vi "Target3.vi"   [LabVIEW 2025]
uses:
  <vilib>/eio/utilities/niEioResolveVilibRelativePath.vi
  <vilib>/rvi/interface/RandomDataEmulation/niFpgaRandomDataHandleErrors.vi
  <vilib>/rvi/Memory/Memory_Emulation/nirvimemoryFastEmulation.vi
  <vilib>/rvi/Memory/Memory_Emulation/nirvimemoryEmulation.vi
  <vilib>/rvi/Emulation/niFpgaEmulationIsFPGAContextNoSignature.vi
  <vilib>/rvi/DataTransferAndStorage/Container/Common/niFpgaContainerGetUniqueNameForEmu.vi
  <vilib>/rvi/Emulation/niFpgaProcessEmulError.vi
  <vilib>/rvi/Emulation/niFpgaSctlEmulationGetInTimedLoop.vi
  <vilib>/rvi/errors/nirviReportUnexpectedCaseInternalError (U32).vi
  <vilib>/rvi/DataTransferAndStorage/Container/XNode/niFpgaContainer.xnode
  <vilib>/rvi/interface/RandomDataEmulation/nirviRandomDataFpgaReadWriteTemplate.vi
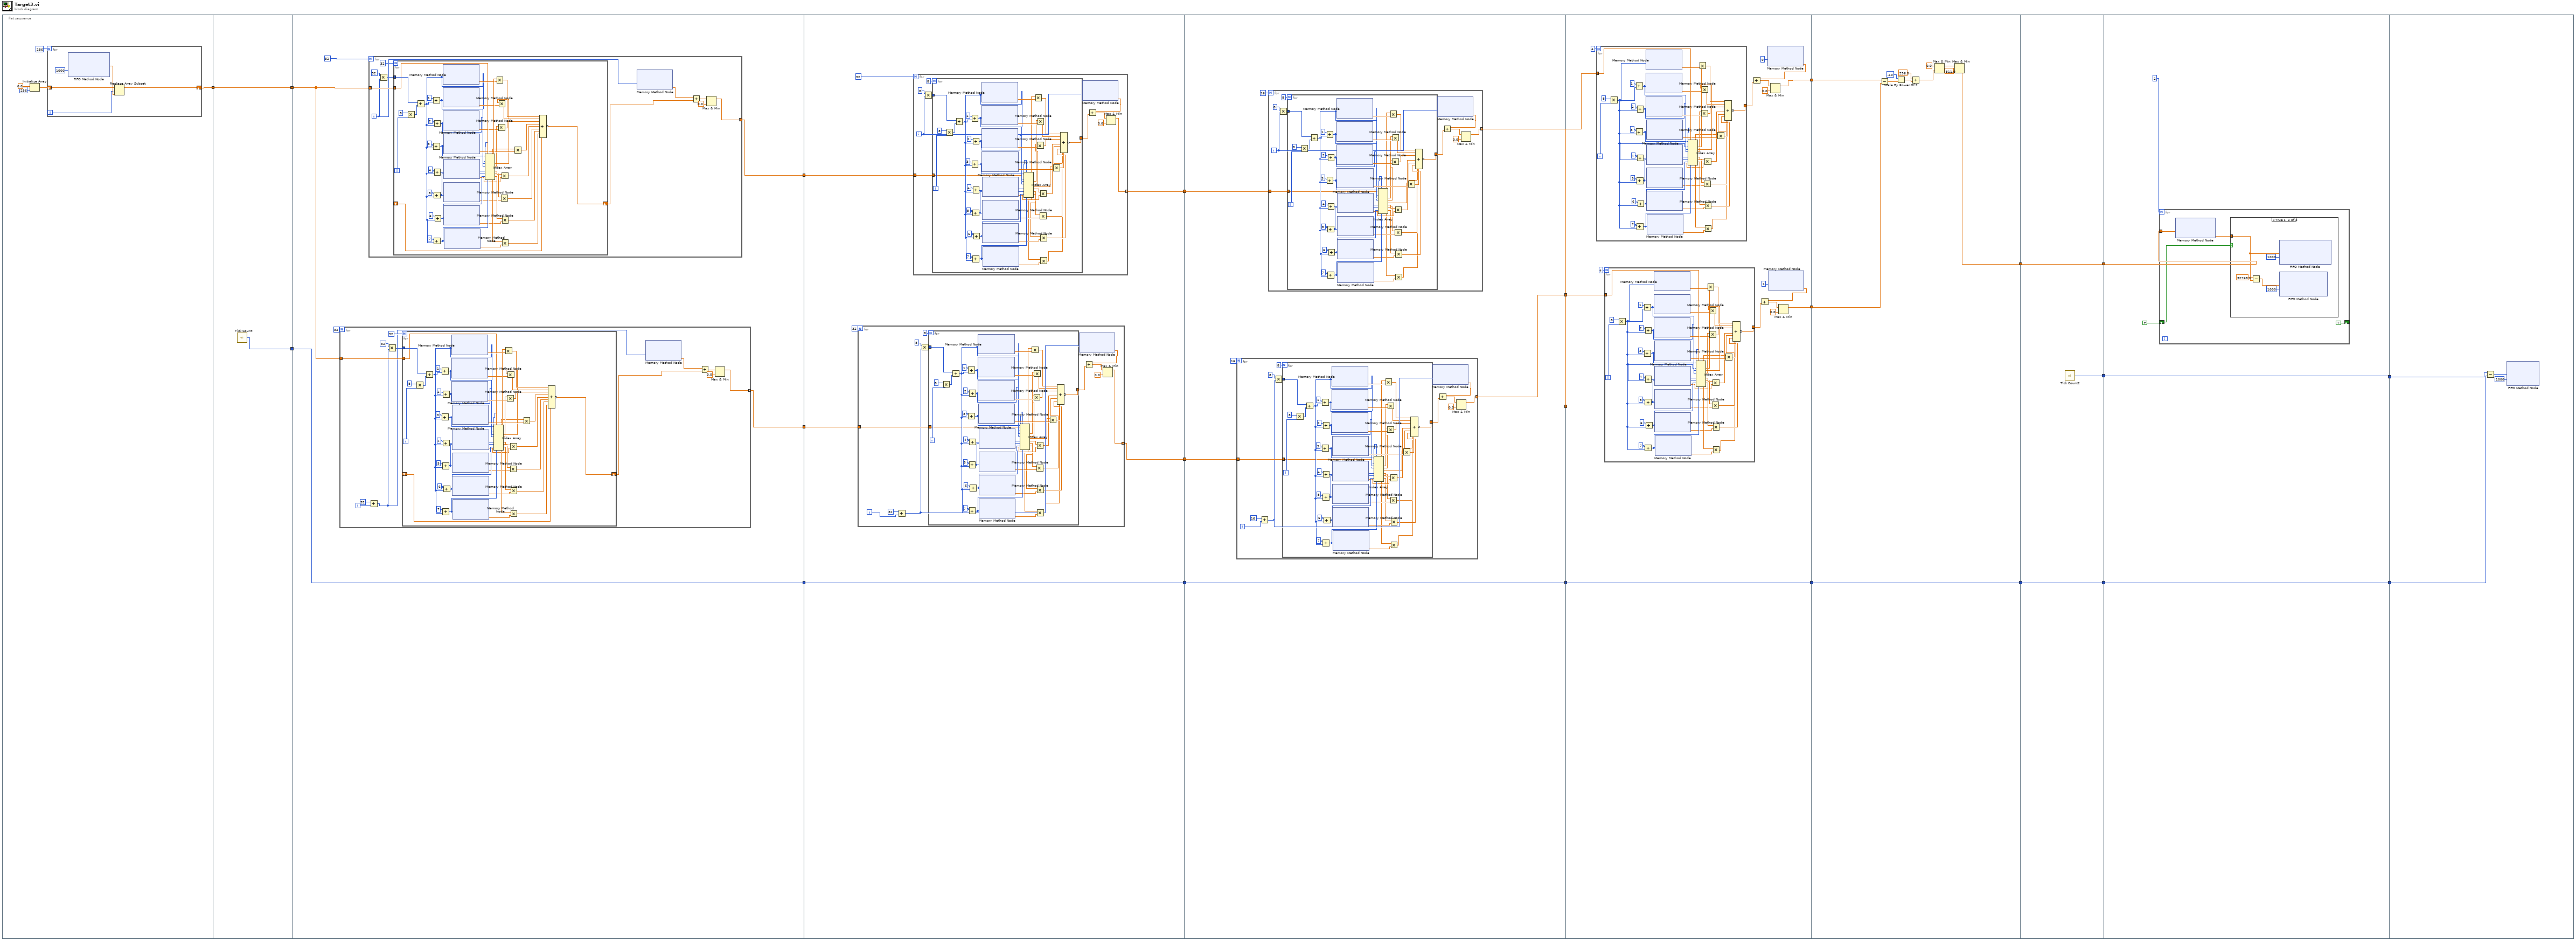
[diagram p0: block diagram]
diagram:
  n1 = flat-sequence {
    tunnel: [w26] -> w22
    tunnel: w22 -> [w34]
    tunnel: [w34] -> w21
    tunnel: [w33] -> w20
    tunnel: w21 -> [w36]
    tunnel: w20 -> [w39]
    tunnel: [w39] -> w10
    tunnel: [w38] -> w9
    tunnel: [w35] -> w2
    tunnel: w10 -> [w161]
    tunnel: [w161] -> w7
    tunnel: w9 -> [w159]
    tunnel: [w158] -> w5
    tunnel: w2 -> [w156]
    tunnel: [w155] -> w1
    tunnel: [w278] -> w8
    tunnel: w7 -> [w280]
    tunnel: [w280] -> w6
    tunnel: w5 -> [w277]
    tunnel: [w276] -> w3
    tunnel: w1 -> [w274]
    tunnel: w8 -> [w408]
    tunnel: [w407] -> w19
    tunnel: [w409] -> w11
    tunnel: w6 -> [w409]
    tunnel: [w394] -> w4
    tunnel: w3 -> [w393]
    tunnel: w19 -> [w496]
    tunnel: [w499] -> w18
    tunnel: [w498] -> w12
    tunnel: w11 -> [w498]
    tunnel: w4 -> [w497]
    tunnel: w18 -> [w510]
    tunnel: [w510] -> w17
    tunnel: [w509] -> w16
    tunnel: [w508] -> w13
    tunnel: w12 -> [w508]
    tunnel: w17 -> [w514]
    tunnel: [w512] -> w15
    tunnel: w16 -> [w512]
    tunnel: [w511] -> w14
    tunnel: w13 -> [w511]
    tunnel: w15 -> [w528]
    tunnel: w14 -> [w525]
    frame #0 {
      n2 = Initialize Array(sgl 0.0 ("element"), 256 ("dimension size")) -> (w23:sgl[])
      n3 = for {
        N: 256 -> [_]
        shift-right: [w29] -> w26
        shift-left: w23 -> [w31]
        i -> [w28]
        n4 = xnode ("FIFO Method Node")("Timeout"=1000) -> ("Element"=w30:sgl)  [unwired: 1 in, 2 out]
        n5 = Replace Array Subset(array=w31, new element=w30, index=w28) -> (w29:sgl[])
      }
    }
    frame #1 {
      n6 = call "Tick Count"() -> ("Tick Count(uSec)"=w33:u32)
    }
    frame #2 {
      n7 = for {
        N: 32 -> [_]
        tunnel: w36 -> [w47]
        tunnel: [w46] -> w35 mode=indexing
        i -> [w43]
        n8 = Add(x=32, y=w43) -> (x+y=w42:i32)
        n9 = Multiply(x=32, y=w42) -> (x*y=w50:i32)
        n10 = for {
          N: 32 -> [_]
          tunnel: w50 -> [w98]
          tunnel: w47 -> [w84]
          shift-right: [w53] -> w45
          shift-left: _ -> [w54]
          i -> [w97]
          n11 = Multiply(x=8, y=w97) -> (x*y=w95:i32)
          n12 = Add(x=w98, y=w95) -> (x+y=w59:i32)
          n13 = Add(x=1, y=w59) -> (x+y=w81:i32)
          n14 = Add(x=3, y=w59) -> (x+y=w77:i32)
          n15 = Add(x=5, y=w59) -> (x+y=w70:i32)
          n16 = Add(x=7, y=w59) -> (x+y=w68:i32)
          n17 = Add(x=2, y=w59) -> (x+y=w76:i32)
          n18 = Add(x=4, y=w59) -> (x+y=w71:i32)
          n19 = Add(x=6, y=w59) -> (x+y=w69:i32)
          n20 = xnode ("Memory Method Node")("Address"=w59) -> ("Data"=w90:sgl)  [unwired: 1 in, 1 out]
          n21 = xnode ("Memory Method Node")("Address"=w81) -> ("Data"=w85:sgl)  [unwired: 1 in, 1 out]
          n22 = xnode ("Memory Method Node")("Address"=w76) -> ("Data"=w82:sgl)  [unwired: 1 in, 1 out]
          n23 = xnode ("Memory Method Node")("Address"=w77) -> ("Data"=w83:sgl)  [unwired: 1 in, 1 out]
          n24 = xnode ("Memory Method Node")("Address"=w71) -> ("Data"=w60:sgl)  [unwired: 1 in, 1 out]
          n25 = xnode ("Memory Method Node")("Address"=w70) -> ("Data"=w61:sgl)  [unwired: 1 in, 1 out]
          n26 = xnode ("Memory Method Node")("Address"=w69) -> ("Data"=w62:sgl)  [unwired: 1 in, 1 out]
          n27 = xnode ("Memory Method Node")("Address"=w68) -> ("Data"=w63:sgl)  [unwired: 1 in, 1 out]
          n28 = Index Array(array=w84, index #1=w59, index #2=w81, index #3=w76, index #4=w77, index #5=w71, index #6=w70, index #7=w69, index #8=w68) -> (element #1=w91:sgl, element #2=w80:sgl, element #3=w79:sgl, element #4=w78:sgl, element #5=w67:sgl, element #6=w66:sgl, element #7=w65:sgl, element #8=w64:sgl)
          n29 = Multiply(x=w91, y=w90) -> (x*y=w89:sgl)
          n30 = Multiply(x=w79, y=w82) -> (x*y=w87:sgl)
          n31 = Multiply(x=w80, y=w85) -> (x*y=w88:sgl)
          n32 = Multiply(x=w66, y=w61) -> (x*y=w57:sgl)
          n33 = Multiply(x=w67, y=w60) -> (x*y=w58:sgl)
          n34 = Multiply(x=w65, y=w62) -> (x*y=w56:sgl)
          n35 = Multiply(x=w64, y=w63) -> (x*y=w55:sgl)
          n36 = Multiply(x=w78, y=w83) -> (x*y=w86:sgl)
          n37 = Compound Arithmetic op=ADD(w89, w88, w87, w86, w58, w57, w56, w55, w54) -> (invert w53:sgl)
        }
        n38 = xnode ("Memory Method Node")("Address"=w42) -> ("Data"=w44:sgl)  [unwired: 1 in, 1 out]
        n39 = Add(x=w44, y=w45) -> (x+y=w49:sgl)
        n40 = Max & Min(x=w49, y=sgl 0.0) -> (max(x,y)=w46:sgl)  [unwired: 1 out]
      }
      n41 = for {
        N: 32 -> [_]
        tunnel: w36 -> [w103]
        tunnel: [w101] -> w38 mode=indexing
        i -> [w102]
        n42 = Multiply(x=32, y=w102) -> (x*y=w106:i32)
        n43 = for {
          N: 32 -> [_]
          tunnel: w106 -> [w154]
          tunnel: w103 -> [w140]
          shift-right: [w109] -> w100
          shift-left: _ -> [w110]
          i -> [w153]
          n44 = Multiply(x=8, y=w153) -> (x*y=w151:i32)
          n45 = Add(x=w154, y=w151) -> (x+y=w115:i32)
          n46 = Add(x=1, y=w115) -> (x+y=w137:i32)
          n47 = Add(x=3, y=w115) -> (x+y=w133:i32)
          n48 = Add(x=5, y=w115) -> (x+y=w126:i32)
          n49 = Add(x=7, y=w115) -> (x+y=w124:i32)
          n50 = Add(x=2, y=w115) -> (x+y=w132:i32)
          n51 = Add(x=4, y=w115) -> (x+y=w127:i32)
          n52 = Add(x=6, y=w115) -> (x+y=w125:i32)
          n53 = xnode ("Memory Method Node")("Address"=w115) -> ("Data"=w146:sgl)  [unwired: 1 in, 1 out]
          n54 = xnode ("Memory Method Node")("Address"=w137) -> ("Data"=w141:sgl)  [unwired: 1 in, 1 out]
          n55 = xnode ("Memory Method Node")("Address"=w132) -> ("Data"=w138:sgl)  [unwired: 1 in, 1 out]
          n56 = xnode ("Memory Method Node")("Address"=w133) -> ("Data"=w139:sgl)  [unwired: 1 in, 1 out]
          n57 = xnode ("Memory Method Node")("Address"=w127) -> ("Data"=w116:sgl)  [unwired: 1 in, 1 out]
          n58 = xnode ("Memory Method Node")("Address"=w126) -> ("Data"=w117:sgl)  [unwired: 1 in, 1 out]
          n59 = xnode ("Memory Method Node")("Address"=w125) -> ("Data"=w118:sgl)  [unwired: 1 in, 1 out]
          n60 = xnode ("Memory Method Node")("Address"=w124) -> ("Data"=w119:sgl)  [unwired: 1 in, 1 out]
          n61 = Index Array(array=w140, index #1=w115, index #2=w137, index #3=w132, index #4=w133, index #5=w127, index #6=w126, index #7=w125, index #8=w124) -> (element #1=w147:sgl, element #2=w136:sgl, element #3=w135:sgl, element #4=w134:sgl, element #5=w123:sgl, element #6=w122:sgl, element #7=w121:sgl, element #8=w120:sgl)
          n62 = Multiply(x=w147, y=w146) -> (x*y=w145:sgl)
          n63 = Multiply(x=w135, y=w138) -> (x*y=w143:sgl)
          n64 = Multiply(x=w136, y=w141) -> (x*y=w144:sgl)
          n65 = Multiply(x=w122, y=w117) -> (x*y=w113:sgl)
          n66 = Multiply(x=w123, y=w116) -> (x*y=w114:sgl)
          n67 = Multiply(x=w121, y=w118) -> (x*y=w112:sgl)
          n68 = Multiply(x=w120, y=w119) -> (x*y=w111:sgl)
          n69 = Multiply(x=w134, y=w139) -> (x*y=w142:sgl)
          n70 = Compound Arithmetic op=ADD(w145, w144, w143, w142, w114, w113, w112, w111, w110) -> (invert w109:sgl)
        }
        n71 = xnode ("Memory Method Node")("Address"=w102) -> ("Data"=w99:sgl)  [unwired: 1 in, 1 out]
        n72 = Add(x=w99, y=w100) -> (x+y=w105:sgl)
        n73 = Max & Min(x=w105, y=sgl 0.0) -> (max(x,y)=w101:sgl)  [unwired: 1 out]
      }
    }
    frame #3 {
      n74 = for {
        N: 32 -> [_]
        tunnel: w156 -> [w166]
        tunnel: [w165] -> w155 mode=indexing
        i -> [w163]
        n75 = Add(x=32, y=w163) -> (x+y=w162:i32)
        n76 = Multiply(x=8, y=w162) -> (x*y=w170:i32)
        n77 = for {
          N: 8 -> [_]
          tunnel: w170 -> [w218]
          tunnel: [w203] -> w167
          tunnel: w166 -> [w182]
          i -> [w217]
          n78 = Multiply(x=8, y=w217) -> (x*y=w215:i32)
          n79 = Add(x=w218, y=w215) -> (x+y=w183:i32)
          n80 = Add(x=1, y=w183) -> (x+y=w202:i32)
          n81 = Add(x=3, y=w183) -> (x+y=w201:i32)
          n82 = Add(x=5, y=w183) -> (x+y=w194:i32)
          n83 = Add(x=7, y=w183) -> (x+y=w192:i32)
          n84 = Add(x=2, y=w183) -> (x+y=w200:i32)
          n85 = Add(x=4, y=w183) -> (x+y=w195:i32)
          n86 = Add(x=6, y=w183) -> (x+y=w193:i32)
          n87 = xnode ("Memory Method Node")("Address"=w183) -> ("Data"=w211:sgl)  [unwired: 1 in, 1 out]
          n88 = xnode ("Memory Method Node")("Address"=w202) -> ("Data"=w206:sgl)  [unwired: 1 in, 1 out]
          n89 = xnode ("Memory Method Node")("Address"=w200) -> ("Data"=w204:sgl)  [unwired: 1 in, 1 out]
          n90 = xnode ("Memory Method Node")("Address"=w201) -> ("Data"=w205:sgl)  [unwired: 1 in, 1 out]
          n91 = xnode ("Memory Method Node")("Address"=w195) -> ("Data"=w188:sgl)  [unwired: 1 in, 1 out]
          n92 = xnode ("Memory Method Node")("Address"=w194) -> ("Data"=w189:sgl)  [unwired: 1 in, 1 out]
          n93 = xnode ("Memory Method Node")("Address"=w193) -> ("Data"=w190:sgl)  [unwired: 1 in, 1 out]
          n94 = xnode ("Memory Method Node")("Address"=w192) -> ("Data"=w191:sgl)  [unwired: 1 in, 1 out]
          n95 = Index Array(array=w182, index #1=w183, index #2=w202, index #3=w200, index #4=w201, index #5=w195, index #6=w194, index #7=w193, index #8=w192) -> (element #1=w181:sgl, element #2=w180:sgl, element #3=w179:sgl, element #4=w177:sgl, element #5=w178:sgl, element #6=w176:sgl, element #7=w175:sgl, element #8=w174:sgl)
          n96 = Multiply(x=w181, y=w211) -> (x*y=w210:sgl)
          n97 = Multiply(x=w179, y=w204) -> (x*y=w208:sgl)
          n98 = Multiply(x=w180, y=w206) -> (x*y=w209:sgl)
          n99 = Multiply(x=w176, y=w189) -> (x*y=w186:sgl)
          n100 = Multiply(x=w178, y=w188) -> (x*y=w187:sgl)
          n101 = Multiply(x=w175, y=w190) -> (x*y=w185:sgl)
          n102 = Multiply(x=w174, y=w191) -> (x*y=w184:sgl)
          n103 = Multiply(x=w177, y=w205) -> (x*y=w207:sgl)
          n104 = Compound Arithmetic op=ADD(w210, w209, w208, w207, w187, w186, w185, w184) -> (invert w203:sgl)
        }
        n105 = xnode ("Memory Method Node")("Address"=w162) -> ("Data"=w172:sgl)  [unwired: 1 in, 1 out]
        n106 = Add(x=w172, y=w167) -> (x+y=w169:sgl)
        n107 = Max & Min(x=w169, y=sgl 0.0) -> (max(x,y)=w165:sgl)  [unwired: 1 out]
      }
      n108 = for {
        N: 32 -> [_]
        tunnel: w159 -> [w220]
        tunnel: [w219] -> w158 mode=indexing
        i -> [w225]
        n109 = Multiply(x=8, y=w225) -> (x*y=w224:i32)
        n110 = for {
          N: 8 -> [_]
          tunnel: w224 -> [w273]
          tunnel: [w258] -> w221
          tunnel: w220 -> [w237]
          i -> [w272]
          n111 = Multiply(x=8, y=w272) -> (x*y=w270:i32)
          n112 = Add(x=w273, y=w270) -> (x+y=w238:i32)
          n113 = Add(x=1, y=w238) -> (x+y=w257:i32)
          n114 = Add(x=3, y=w238) -> (x+y=w256:i32)
          n115 = Add(x=5, y=w238) -> (x+y=w249:i32)
          n116 = Add(x=7, y=w238) -> (x+y=w247:i32)
          n117 = Add(x=2, y=w238) -> (x+y=w255:i32)
          n118 = Add(x=4, y=w238) -> (x+y=w250:i32)
          n119 = Add(x=6, y=w238) -> (x+y=w248:i32)
          n120 = xnode ("Memory Method Node")("Address"=w238) -> ("Data"=w266:sgl)  [unwired: 1 in, 1 out]
          n121 = xnode ("Memory Method Node")("Address"=w257) -> ("Data"=w261:sgl)  [unwired: 1 in, 1 out]
          n122 = xnode ("Memory Method Node")("Address"=w255) -> ("Data"=w259:sgl)  [unwired: 1 in, 1 out]
          n123 = xnode ("Memory Method Node")("Address"=w256) -> ("Data"=w260:sgl)  [unwired: 1 in, 1 out]
          n124 = xnode ("Memory Method Node")("Address"=w250) -> ("Data"=w243:sgl)  [unwired: 1 in, 1 out]
          n125 = xnode ("Memory Method Node")("Address"=w249) -> ("Data"=w244:sgl)  [unwired: 1 in, 1 out]
          n126 = xnode ("Memory Method Node")("Address"=w248) -> ("Data"=w245:sgl)  [unwired: 1 in, 1 out]
          n127 = xnode ("Memory Method Node")("Address"=w247) -> ("Data"=w246:sgl)  [unwired: 1 in, 1 out]
          n128 = Index Array(array=w237, index #1=w238, index #2=w257, index #3=w255, index #4=w256, index #5=w250, index #6=w249, index #7=w248, index #8=w247) -> (element #1=w236:sgl, element #2=w235:sgl, element #3=w234:sgl, element #4=w232:sgl, element #5=w233:sgl, element #6=w231:sgl, element #7=w230:sgl, element #8=w229:sgl)
          n129 = Multiply(x=w236, y=w266) -> (x*y=w265:sgl)
          n130 = Multiply(x=w234, y=w259) -> (x*y=w263:sgl)
          n131 = Multiply(x=w235, y=w261) -> (x*y=w264:sgl)
          n132 = Multiply(x=w231, y=w244) -> (x*y=w241:sgl)
          n133 = Multiply(x=w233, y=w243) -> (x*y=w242:sgl)
          n134 = Multiply(x=w230, y=w245) -> (x*y=w240:sgl)
          n135 = Multiply(x=w229, y=w246) -> (x*y=w239:sgl)
          n136 = Multiply(x=w232, y=w260) -> (x*y=w262:sgl)
          n137 = Compound Arithmetic op=ADD(w265, w264, w263, w262, w242, w241, w240, w239) -> (invert w258:sgl)
        }
        n138 = xnode ("Memory Method Node")("Address"=w225) -> ("Data"=w227:sgl)  [unwired: 1 in, 1 out]
        n139 = Add(x=w227, y=w221) -> (x+y=w223:sgl)
        n140 = Max & Min(x=w223, y=sgl 0.0) -> (max(x,y)=w219:sgl)  [unwired: 1 out]
      }
    }
    frame #4 {
      n141 = for {
        N: 16 -> [_]
        tunnel: [w286] -> w276 mode=indexing
        tunnel: w274 -> [w284]
        i -> [w281]
        n142 = Add(x=16, y=w281) -> (x+y=w282:i32)
        n143 = Multiply(x=8, y=w282) -> (x*y=w289:i32)
        n144 = for {
          N: 8 -> [_]
          tunnel: w289 -> [w337]
          tunnel: [w322] -> w285
          tunnel: w284 -> [w301]
          i -> [w336]
          n145 = Multiply(x=8, y=w336) -> (x*y=w334:i32)
          n146 = Add(x=w337, y=w334) -> (x+y=w302:i32)
          n147 = Add(x=1, y=w302) -> (x+y=w321:i32)
          n148 = Add(x=3, y=w302) -> (x+y=w320:i32)
          n149 = Add(x=5, y=w302) -> (x+y=w313:i32)
          n150 = Add(x=7, y=w302) -> (x+y=w311:i32)
          n151 = Add(x=2, y=w302) -> (x+y=w319:i32)
          n152 = Add(x=4, y=w302) -> (x+y=w314:i32)
          n153 = Add(x=6, y=w302) -> (x+y=w312:i32)
          n154 = xnode ("Memory Method Node")("Address"=w302) -> ("Data"=w330:sgl)  [unwired: 1 in, 1 out]
          n155 = xnode ("Memory Method Node")("Address"=w321) -> ("Data"=w325:sgl)  [unwired: 1 in, 1 out]
          n156 = xnode ("Memory Method Node")("Address"=w319) -> ("Data"=w323:sgl)  [unwired: 1 in, 1 out]
          n157 = xnode ("Memory Method Node")("Address"=w320) -> ("Data"=w324:sgl)  [unwired: 1 in, 1 out]
          n158 = xnode ("Memory Method Node")("Address"=w314) -> ("Data"=w307:sgl)  [unwired: 1 in, 1 out]
          n159 = xnode ("Memory Method Node")("Address"=w313) -> ("Data"=w308:sgl)  [unwired: 1 in, 1 out]
          n160 = xnode ("Memory Method Node")("Address"=w312) -> ("Data"=w309:sgl)  [unwired: 1 in, 1 out]
          n161 = xnode ("Memory Method Node")("Address"=w311) -> ("Data"=w310:sgl)  [unwired: 1 in, 1 out]
          n162 = Index Array(array=w301, index #1=w302, index #2=w321, index #3=w319, index #4=w320, index #5=w314, index #6=w313, index #7=w312, index #8=w311) -> (element #1=w300:sgl, element #2=w299:sgl, element #3=w298:sgl, element #4=w297:sgl, element #5=w296:sgl, element #6=w295:sgl, element #7=w294:sgl, element #8=w293:sgl)
          n163 = Multiply(x=w300, y=w330) -> (x*y=w329:sgl)
          n164 = Multiply(x=w298, y=w323) -> (x*y=w327:sgl)
          n165 = Multiply(x=w299, y=w325) -> (x*y=w328:sgl)
          n166 = Multiply(x=w295, y=w308) -> (x*y=w305:sgl)
          n167 = Multiply(x=w296, y=w307) -> (x*y=w306:sgl)
          n168 = Multiply(x=w294, y=w309) -> (x*y=w304:sgl)
          n169 = Multiply(x=w293, y=w310) -> (x*y=w303:sgl)
          n170 = Multiply(x=w297, y=w324) -> (x*y=w326:sgl)
          n171 = Compound Arithmetic op=ADD(w329, w328, w327, w326, w306, w305, w304, w303) -> (invert w322:sgl)
        }
        n172 = xnode ("Memory Method Node")("Address"=w282) -> ("Data"=w291:sgl)  [unwired: 1 in, 1 out]
        n173 = Add(x=w291, y=w285) -> (x+y=w288:sgl)
        n174 = Max & Min(x=w288, y=sgl 0.0) -> (max(x,y)=w286:sgl)  [unwired: 1 out]
      }
      n175 = for {
        N: 16 -> [_]
        tunnel: [w340] -> w278 mode=indexing
        tunnel: w277 -> [w338]
        i -> [w344]
        n176 = Multiply(x=8, y=w344) -> (x*y=w343:i32)
        n177 = for {
          N: 8 -> [_]
          tunnel: w343 -> [w392]
          tunnel: [w377] -> w339
          tunnel: w338 -> [w356]
          i -> [w391]
          n178 = Multiply(x=8, y=w391) -> (x*y=w389:i32)
          n179 = Add(x=w392, y=w389) -> (x+y=w357:i32)
          n180 = Add(x=1, y=w357) -> (x+y=w376:i32)
          n181 = Add(x=3, y=w357) -> (x+y=w375:i32)
          n182 = Add(x=5, y=w357) -> (x+y=w368:i32)
          n183 = Add(x=7, y=w357) -> (x+y=w366:i32)
          n184 = Add(x=2, y=w357) -> (x+y=w374:i32)
          n185 = Add(x=4, y=w357) -> (x+y=w369:i32)
          n186 = Add(x=6, y=w357) -> (x+y=w367:i32)
          n187 = xnode ("Memory Method Node")("Address"=w357) -> ("Data"=w385:sgl)  [unwired: 1 in, 1 out]
          n188 = xnode ("Memory Method Node")("Address"=w376) -> ("Data"=w380:sgl)  [unwired: 1 in, 1 out]
          n189 = xnode ("Memory Method Node")("Address"=w374) -> ("Data"=w378:sgl)  [unwired: 1 in, 1 out]
          n190 = xnode ("Memory Method Node")("Address"=w375) -> ("Data"=w379:sgl)  [unwired: 1 in, 1 out]
          n191 = xnode ("Memory Method Node")("Address"=w369) -> ("Data"=w362:sgl)  [unwired: 1 in, 1 out]
          n192 = xnode ("Memory Method Node")("Address"=w368) -> ("Data"=w363:sgl)  [unwired: 1 in, 1 out]
          n193 = xnode ("Memory Method Node")("Address"=w367) -> ("Data"=w364:sgl)  [unwired: 1 in, 1 out]
          n194 = xnode ("Memory Method Node")("Address"=w366) -> ("Data"=w365:sgl)  [unwired: 1 in, 1 out]
          n195 = Index Array(array=w356, index #1=w357, index #2=w376, index #3=w374, index #4=w375, index #5=w369, index #6=w368, index #7=w367, index #8=w366) -> (element #1=w355:sgl, element #2=w354:sgl, element #3=w353:sgl, element #4=w352:sgl, element #5=w351:sgl, element #6=w350:sgl, element #7=w349:sgl, element #8=w348:sgl)
          n196 = Multiply(x=w355, y=w385) -> (x*y=w384:sgl)
          n197 = Multiply(x=w353, y=w378) -> (x*y=w382:sgl)
          n198 = Multiply(x=w354, y=w380) -> (x*y=w383:sgl)
          n199 = Multiply(x=w350, y=w363) -> (x*y=w360:sgl)
          n200 = Multiply(x=w351, y=w362) -> (x*y=w361:sgl)
          n201 = Multiply(x=w349, y=w364) -> (x*y=w359:sgl)
          n202 = Multiply(x=w348, y=w365) -> (x*y=w358:sgl)
          n203 = Multiply(x=w352, y=w379) -> (x*y=w381:sgl)
          n204 = Compound Arithmetic op=ADD(w384, w383, w382, w381, w361, w360, w359, w358) -> (invert w377:sgl)
        }
        n205 = xnode ("Memory Method Node")("Address"=w344) -> ("Data"=w346:sgl)  [unwired: 1 in, 1 out]
        n206 = Add(x=w346, y=w339) -> (x+y=w342:sgl)
        n207 = Max & Min(x=w342, y=sgl 0.0) -> (max(x,y)=w340:sgl)  [unwired: 1 out]
      }
    }
    frame #5 {
      n208 = for {
        N: 4 -> [_]
        tunnel: w408 -> [w483]
        tunnel: [w480] -> w402
        i -> [w495]
        n209 = Multiply(x=8, y=w495) -> (x*y=w453:i32)
        n210 = Add(x=1, y=w453) -> (x+y=w479:i32)
        n211 = Add(x=3, y=w453) -> (x+y=w475:i32)
        n212 = Add(x=5, y=w453) -> (x+y=w468:i32)
        n213 = Add(x=7, y=w453) -> (x+y=w466:i32)
        n214 = Add(x=2, y=w453) -> (x+y=w474:i32)
        n215 = Add(x=4, y=w453) -> (x+y=w469:i32)
        n216 = Add(x=6, y=w453) -> (x+y=w467:i32)
        n217 = xnode ("Memory Method Node")("Address"=w453) -> ("Data"=w489:sgl)  [unwired: 1 in, 1 out]
        n218 = xnode ("Memory Method Node")("Address"=w479) -> ("Data"=w484:sgl)  [unwired: 1 in, 1 out]
        n219 = xnode ("Memory Method Node")("Address"=w474) -> ("Data"=w481:sgl)  [unwired: 1 in, 1 out]
        n220 = xnode ("Memory Method Node")("Address"=w475) -> ("Data"=w482:sgl)  [unwired: 1 in, 1 out]
        n221 = xnode ("Memory Method Node")("Address"=w469) -> ("Data"=w458:sgl)  [unwired: 1 in, 1 out]
        n222 = xnode ("Memory Method Node")("Address"=w468) -> ("Data"=w459:sgl)  [unwired: 1 in, 1 out]
        n223 = xnode ("Memory Method Node")("Address"=w467) -> ("Data"=w460:sgl)  [unwired: 1 in, 1 out]
        n224 = xnode ("Memory Method Node")("Address"=w466) -> ("Data"=w461:sgl)  [unwired: 1 in, 1 out]
        n225 = Index Array(array=w483, index #1=w453, index #2=w479, index #3=w474, index #4=w475, index #5=w469, index #6=w468, index #7=w467, index #8=w466) -> (element #1=w490:sgl, element #2=w478:sgl, element #3=w477:sgl, element #4=w476:sgl, element #5=w465:sgl, element #6=w464:sgl, element #7=w463:sgl, element #8=w462:sgl)
        n226 = Multiply(x=w490, y=w489) -> (x*y=w488:sgl)
        n227 = Multiply(x=w477, y=w481) -> (x*y=w486:sgl)
        n228 = Multiply(x=w478, y=w484) -> (x*y=w487:sgl)
        n229 = Multiply(x=w464, y=w459) -> (x*y=w456:sgl)
        n230 = Multiply(x=w465, y=w458) -> (x*y=w457:sgl)
        n231 = Multiply(x=w463, y=w460) -> (x*y=w455:sgl)
        n232 = Multiply(x=w462, y=w461) -> (x*y=w454:sgl)
        n233 = Multiply(x=w476, y=w482) -> (x*y=w485:sgl)
        n234 = Compound Arithmetic op=ADD(w488, w487, w486, w485, w457, w456, w455, w454) -> (invert w480:sgl)
      }
      n235 = for {
        N: 4 -> [_]
        tunnel: w393 -> [w440]
        tunnel: [w437] -> w397
        i -> [w452]
        n236 = Multiply(x=8, y=w452) -> (x*y=w410:i32)
        n237 = Add(x=1, y=w410) -> (x+y=w436:i32)
        n238 = Add(x=3, y=w410) -> (x+y=w432:i32)
        n239 = Add(x=5, y=w410) -> (x+y=w425:i32)
        n240 = Add(x=7, y=w410) -> (x+y=w423:i32)
        n241 = Add(x=2, y=w410) -> (x+y=w431:i32)
        n242 = Add(x=4, y=w410) -> (x+y=w426:i32)
        n243 = Add(x=6, y=w410) -> (x+y=w424:i32)
        n244 = xnode ("Memory Method Node")("Address"=w410) -> ("Data"=w446:sgl)  [unwired: 1 in, 1 out]
        n245 = xnode ("Memory Method Node")("Address"=w436) -> ("Data"=w441:sgl)  [unwired: 1 in, 1 out]
        n246 = xnode ("Memory Method Node")("Address"=w431) -> ("Data"=w438:sgl)  [unwired: 1 in, 1 out]
        n247 = xnode ("Memory Method Node")("Address"=w432) -> ("Data"=w439:sgl)  [unwired: 1 in, 1 out]
        n248 = xnode ("Memory Method Node")("Address"=w426) -> ("Data"=w415:sgl)  [unwired: 1 in, 1 out]
        n249 = xnode ("Memory Method Node")("Address"=w425) -> ("Data"=w416:sgl)  [unwired: 1 in, 1 out]
        n250 = xnode ("Memory Method Node")("Address"=w424) -> ("Data"=w417:sgl)  [unwired: 1 in, 1 out]
        n251 = xnode ("Memory Method Node")("Address"=w423) -> ("Data"=w418:sgl)  [unwired: 1 in, 1 out]
        n252 = Index Array(array=w440, index #1=w410, index #2=w436, index #3=w431, index #4=w432, index #5=w426, index #6=w425, index #7=w424, index #8=w423) -> (element #1=w447:sgl, element #2=w435:sgl, element #3=w434:sgl, element #4=w433:sgl, element #5=w422:sgl, element #6=w421:sgl, element #7=w420:sgl, element #8=w419:sgl)
        n253 = Multiply(x=w447, y=w446) -> (x*y=w445:sgl)
        n254 = Multiply(x=w434, y=w438) -> (x*y=w443:sgl)
        n255 = Multiply(x=w435, y=w441) -> (x*y=w444:sgl)
        n256 = Multiply(x=w421, y=w416) -> (x*y=w413:sgl)
        n257 = Multiply(x=w422, y=w415) -> (x*y=w414:sgl)
        n258 = Multiply(x=w420, y=w417) -> (x*y=w412:sgl)
        n259 = Multiply(x=w419, y=w418) -> (x*y=w411:sgl)
        n260 = Multiply(x=w433, y=w439) -> (x*y=w442:sgl)
        n261 = Compound Arithmetic op=ADD(w445, w444, w443, w442, w414, w413, w412, w411) -> (invert w437:sgl)
      }
      n262 = xnode ("Memory Method Node")("Address"=u32 0) -> ("Data"=w405:sgl)  [unwired: 1 in, 1 out]
      n263 = Add(x=w405, y=w402) -> (x+y=w404:sgl)
      n264 = xnode ("Memory Method Node")("Address"=u32 1) -> ("Data"=w400:sgl)  [unwired: 1 in, 1 out]
      n265 = Add(x=w400, y=w397) -> (x+y=w399:sgl)
      n266 = Max & Min(x=w404, y=sgl 0.0) -> (max(x,y)=w407:sgl)  [unwired: 1 out]
      n267 = Max & Min(x=w399, y=sgl 0.0) -> (max(x,y)=w394:sgl)  [unwired: 1 out]
    }
    frame #6 {
      n268 = Subtract(x=w496, y=w497) -> (x-y=w504:sgl)
      n269 = Scale By Power Of 2(n=i16 -10, x=w504) -> (x*2^n=w505:sgl)
      n270 = Add(x=sgl 256.0, y=w505) -> (x+y=w506:sgl)
      n271 = Max & Min(x=sgl 0.0, y=w506) -> (max(x,y)=w507:sgl)  [unwired: 1 out]
      n272 = Max & Min(x=w507, y=sgl 511.0) -> (min(x,y)=w499:sgl)  [unwired: 1 out]
    }
    frame #7 {
      n273 = call "Tick Count2"() -> ("Tick Count(uSec)"=w509:u32)
    }
    frame #8 {
      n274 = for {
        N: 2 -> [_]
        tunnel: w514 -> [w519]
        shift-right: [TRUE] -> _
        shift-left: FALSE -> [w518]
        n275 = xnode ("Memory Method Node")("Address"=w519) -> ("Data"=w516:sgl)  [unwired: 1 in, 1 out]
        n276 = case shown="True" w518 {
          tunnel: w516 -> [_ w520]
          frame False {
          }
          frame True {
            n277 = Subtract(x=sgl 32768.0, y=w520) -> (x-y=w524:sgl)
            n278 = xnode ("FIFO Method Node")("Element"=w520, "Timeout"=1000) -> ()  [unwired: 1 in, 2 out]
            n279 = xnode ("FIFO Method Node")("Element"=w524, "Timeout"=1000) -> ()  [unwired: 1 in, 2 out]
          }
        }
      }
    }
    frame #9 {
      n280 = Subtract(x=w528, y=w525) -> (x-y=w527:u32)
      n281 = xnode ("FIFO Method Node")("Element"=w527, "Timeout"=1000) -> ()  [unwired: 1 in, 2 out]
    }
  }
